vi "Stream Communication.vi"() -> ()   [LabVIEW 2018]
uses:
  Stream/Stream.lvclass
  RxTx/RxTx.lvclass
  Stream/Stream.lvclass/Stream.ctl
panel:
  out "error out 2":errorcluster
  out "error out":errorcluster
  in  "RxTx in 2":refnum<class "RxTx.lvclass">
  in  "RxTx in":refnum<class "RxTx.lvclass">
  in  "Stream in 2":refnum<class "Stream.lvclass">
  in  "Stream in":refnum<class "Stream.lvclass">
  # "Filter Wheel Communication System"
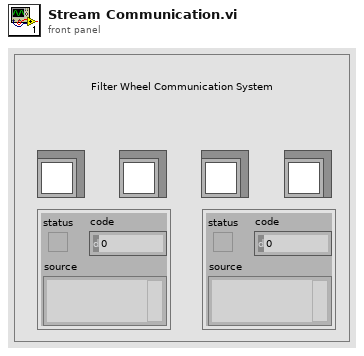
[diagram p1: front panel]
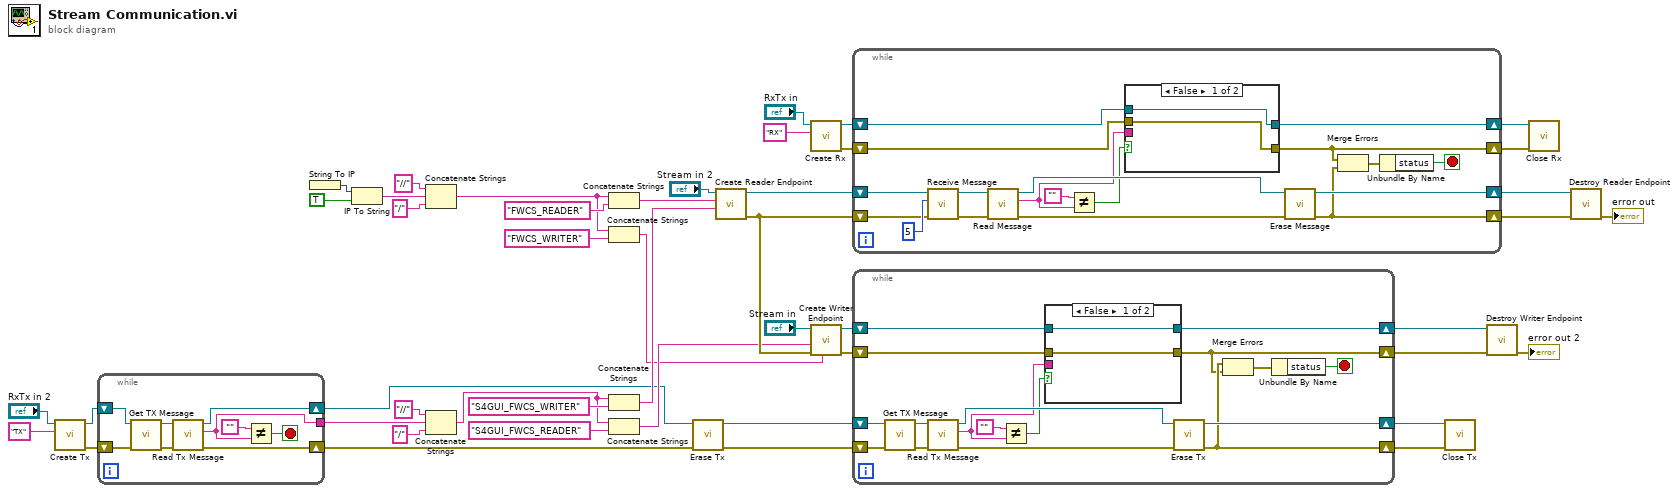
[diagram p0: block diagram]
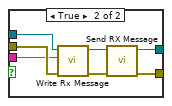
[diagram p2: hidden frame]
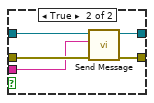
[diagram p3: hidden frame]
diagram:
  n1 = call "Create Tx.vi"("Writer Name"="TX" ("Reader Name"), "RxTx in"="RxTx in 2") -> ("error out"=w6:errorcluster, "RxTx out"=w7:refnum<class "RxTx.lvclass">)  [unwired: 8 in]
  n2 = while {
    shift-right: [w48] -> w4
    shift-left: w7 -> [w51]
    shift-right: [w49] -> w1
    shift-left: w6 -> [w50]
    tunnel: [w47] -> w5
    stop <- w52 stop-if-true
    n3 = call "Get TX Message.vi"("error in (no error)"=w50, "RxTx in"=w51) -> ("error out"=w53:errorcluster, "RxTx out"=w54:refnum<class "RxTx.lvclass">)  [unwired: 8 in]
    n4 = call "Read Tx Message.vi"("error in (no error)"=w53, "RxTx in"=w54) -> ("error out"=w49:errorcluster, "Tx Message"=w47:string, "RxTx out"=w48:refnum<class "RxTx.lvclass">)  [unwired: 7 in]
    n5 = Not Equal?(x="", y=w47) -> (x != y?=w52:bool)
  }
  n6 = String To IP() -> (0:w16:u32)  [unwired: 1 in]
  n7 = IP To String(1:TRUE ("dot notation? (F)"), 2:w16) -> (0:w13:string)
  n8 = Concatenate Strings("//" ("string"), w13, "/" ("string")) -> (w9:string)
  n9 = Concatenate Strings("//" ("string"), w5, "/" ("string")) -> (w8:string)
  n10 = Concatenate Strings(w9, "FWCS_READER" ("Reader Name")) -> (w19:string)
  n11 = Concatenate Strings(w9, "FWCS_WRITER" ("reader name")) -> (w21:string)
  n12 = Concatenate Strings(w8, "S4GUI_FWCS_WRITER" ("reader name")) -> (w25:string)
  n13 = Concatenate Strings(w8, "S4GUI_FWCS_READER" ("Reader Name")) -> (w23:string)
  n14 = call "Erase Tx.vi"("error in (no error)"=w1, "RxTx in"=w4) -> ("error out"=w2:errorcluster, "RxTx out"=w3:refnum<class "RxTx.lvclass">)  [unwired: 8 in]
  n15 = call "Create Reader Endpoint.vi"("writer name"=w25, "reader name"=w19, "Stream in"="Stream in 2") -> ("error out"=w33:errorcluster, "Stream out"=w46:refnum<class "Stream.lvclass">)  [unwired: 7 in]
  n16 = call "Create Rx.vi"("Reader Name"="RX", "RxTx in"="RxTx in") -> ("error out"=w42:errorcluster, "RxTx out"=w43:refnum<class "RxTx.lvclass">)  [unwired: 8 in]
  n17 = call "Create Writer Endpoint.vi"("writer name"=w21, "error in (no error)"=w33, "reader name"=w23, "Stream in"="Stream in") -> ("error out"=w39:errorcluster, "Stream out"=w38:refnum<class "Stream.lvclass">)  [unwired: 6 in]
  n18 = while {
    shift-right: [w66] -> w44
    shift-left: w46 -> [w70]
    shift-right: [w57] -> w45
    shift-left: w33 -> [w69]
    shift-right: [w63] -> w40
    shift-left: w43 -> [w65]
    shift-right: [w56] -> w41
    shift-left: w42 -> [w64]
    stop <- w61 stop-if-true
    n19 = call "Receive Message.vi"("error in (no error)"=w69, "timeout ms"=5, "Stream in"=w70) -> ("error out"=w72:errorcluster, "Stream out"=w71:refnum<class "Stream.lvclass">)  [unwired: 7 in]
    n20 = call "Read Message.vi"("error in (no error)"=w72, "Stream in"=w71) -> ("error out"=w67:errorcluster, "Message"=w58:string, "Stream out"=w68:refnum<class "Stream.lvclass">)  [unwired: 7 in]
    n21 = Not Equal?(x="", y=w58) -> (x != y?=w60:bool)
    n22 = case shown="False" w60 {
      tunnel: w65 -> [w75 w82]
      tunnel: w64 -> [w74 w81]
      tunnel: [w75 w78] -> w63
      tunnel: [w74 w77] -> w56
      tunnel: w58 -> [_ w76]
      frame False {
      }
      frame True {
        n23 = call "Write Rx Message.vi"("error in (no error)"=w81, "Rx Message"=w76, "RxTx in"=w82) -> ("error out"=w80:errorcluster, "RxTx out"=w79:refnum<class "RxTx.lvclass">)  [unwired: 7 in]
        n24 = call "Send RX Message.vi"("error in (no error)"=w80, "RxTx in"=w79) -> ("error out"=w77:errorcluster, "RxTx out"=w78:refnum<class "RxTx.lvclass">)  [unwired: 8 in]
      }
    }
    n25 = call "Erase Message.vi"("error in (no error)"=w67, "Stream in"=w68) -> ("error out"=w57:errorcluster, "Stream out"=w66:refnum<class "Stream.lvclass">)  [unwired: 8 in]
    n26 = Merge Errors(w56, w57) -> (w62:errorcluster)
    n27 = Unbundle By Name(w62) -> ("status"=w61:bool)
  }
  n28 = while {
    shift-right: [w85] -> w37
    shift-left: w39 -> [w92]
    shift-right: [w90] -> w36
    shift-left: w38 -> [w91]
    shift-right: [w89] -> w34
    shift-left: w3 -> [w87]
    shift-right: [w86] -> w35
    shift-left: w2 -> [w88]
    stop <- w83 stop-if-true
    n29 = call "Get TX Message.vi"("error in (no error)"=w88, "RxTx in"=w87) -> ("error out"=w99:errorcluster, "RxTx out"=w98:refnum<class "RxTx.lvclass">)  [unwired: 8 in]
    n30 = call "Read Tx Message.vi"("error in (no error)"=w99, "RxTx in"=w98) -> ("error out"=w97:errorcluster, "Tx Message"=w94:string, "RxTx out"=w96:refnum<class "RxTx.lvclass">)  [unwired: 7 in]
    n31 = Not Equal?(x="", y=w94) -> (x != y?=w95:bool)
    n32 = case shown="False" w95 {
      tunnel: w91 -> [w101 w106]
      tunnel: w92 -> [w100 w105]
      tunnel: [w100 w104] -> w85
      tunnel: [w101 w103] -> w90
      tunnel: w94 -> [_ w102]
      frame False {
      }
      frame True {
        n33 = call "Send Message.vi"("error in (no error)"=w105, "Message"=w102, "Stream in"=w106) -> ("error out"=w104:errorcluster, "Stream out"=w103:refnum<class "Stream.lvclass">)  [unwired: 7 in]
      }
    }
    n34 = call "Erase Tx.vi"("error in (no error)"=w97, "RxTx in"=w96) -> ("error out"=w86:errorcluster, "RxTx out"=w89:refnum<class "RxTx.lvclass">)  [unwired: 8 in]
    n35 = Merge Errors(w86, w85) -> (w84:errorcluster)
    n36 = Unbundle By Name(w84) -> ("status"=w83:bool)
  }
  n37 = call "Close Tx.vi"("error in (no error)"=w35, "RxTx in"=w34) -> ()  [unwired: 8 in, 2 out]
  n38 = call "Destroy Writer Endpoint.vi"("error in (no error)"=w37, "Stream in"=w36) -> ("error out"=→"error out 2":errorcluster)  [unwired: 8 in, 1 out]
  n39 = call "Close Rx.vi"("error in (no error)"=w41, "RxTx in"=w40) -> ()  [unwired: 8 in, 2 out]
  n40 = call "Destroy Reader Endpoint.vi"("error in (no error)"=w45, "Stream in"=w44) -> ("error out"=→"error out":errorcluster)  [unwired: 8 in, 1 out]
